vi "Check_Reserved_Lines.vi"(8 "error in (no error)":errorcluster, 9 "Controlled Channels":bool[](array[boolean]), 11 "Master Device in":refnum<class "Master Device.lvclass">) -> (0 "error out":errorcluster, 3 "Master Device out":refnum<class "Master Device.lvclass">)   [LabVIEW 2013, in "Master Device.lvclass"]
uses:
  Master Device.lvclass
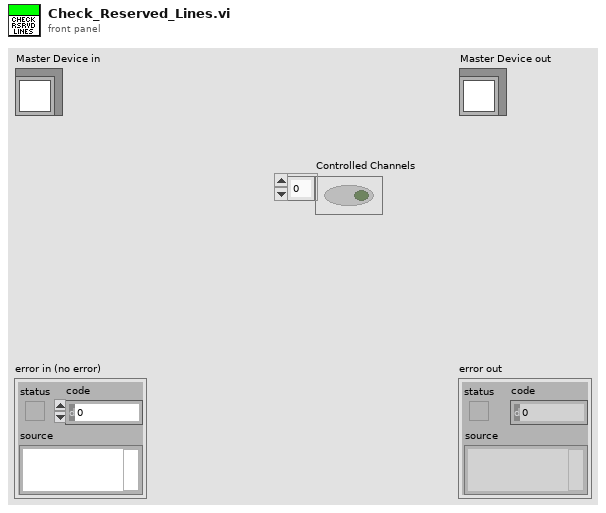
[diagram p1: front panel]
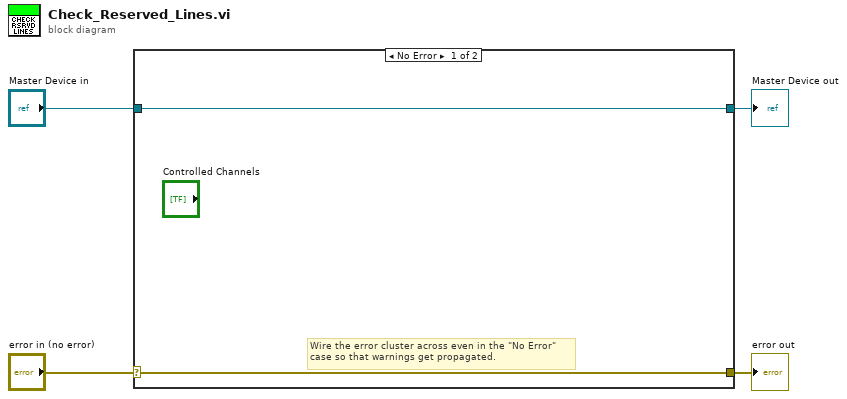
[diagram p0: block diagram]
diagram:
  n1 = case shown="No Error" "error in (no error)" {
    selector: "error in (no error)" -> [w5 w8]
    tunnel: [w5 w8] -> w3
    tunnel: [w6 w7] -> w1
    tunnel: "Master Device in" -> [w6 w7]
    frame No Error {
      # "Wire the error cluster across even in the \"No Error\"\ncase so that warnings get propagated."
    }
    frame Error {
    }
  }
  "error out" <- w3
  "Master Device out" <- w1
